vi "KE622x -- Delta Meas Example.vi"() -> ()   [LabVIEW 2010, in "Keithley 622x.lvlib"]
doc: "Example VI that shows how to perform a 'Delta' measurement. This VI requires both a 622x and a 2182/2182A nano-voltmeter."
uses:
  Keithley 622x.lvlib
  <instrlib>/Keithley 622x LV 2009/Configure/2182 -A/Low Level/Typedefs/KE2182 -- Voltage Ranges.ctl
  <instrlib>/Keithley 622x LV 2009/Configure/2182 -A/Low Level/Typedefs/KE2182 -- NPLCs.ctl
  <instrlib>/Keithley 622x LV 2009/Configure/2182 -A/Low Level/Typedefs/KE2182 -- Filter Type.ctl
  <instrlib>/Keithley 622x LV 2009/Configure/2182 -A/Low Level/Typedefs/KE2182 -- Filter Count.ctl
  <instrlib>/Keithley 622x LV 2009/Configure/2182 -A/Low Level/Typedefs/KE2182 -- Filter Window.ctl
  Configure/Delta PDelta DCon Modes/Low Level/Typedefs/KE622x -- Delta DCon Mode Delay.ctl
  Configure/Delta PDelta DCon Modes/Low Level/Typedefs/KE622x -- Delta PDelta Mode High Level.ctl
  Configure/Delta PDelta DCon Modes/Low Level/Typedefs/KE622x -- Delta PDelta Mode Low Level.ctl
  Configure/Delta PDelta DCon Modes/Low Level/Typedefs/KE622x -- Delta PDelta Mode Num Cycles.ctl
  Configure/Delta PDelta DCon Modes/Low Level/Typedefs/KE622x -- Delta PDelta Mode Num Cycles Mode.ctl
  Configure/Delta PDelta DCon Modes/Typedefs/KE622x -- Delta Mode Params.ctl
  Configure/Units/Typedefs/KE622x -- Voltage Meas Units.ctl
  Configure/Format/Typedefs/KE622x -- Optional Meas Elements.ctl
  Configure/Format/Typedefs/KE622x -- Results Format.ctl
panel:
  out "error out":errorcluster
  in  "Tab Control":enum32{"Results Table", "Plot"}(tab)
  out "Results Table":string[][](table)
  out "Plot":sgl[](graph)
  in  "Results Format":T1={"Results Format"=enum."Single Prec Bin", "Bin Byte Order"=enum."Swapped"}
  in  "Meas Elements To Return":T2={"Timstamp?"=TRUE, "Reading Num?"=TRUE, "Source Value?"=TRUE, "Compliance?"=TRUE, "Average Voltage?"=TRUE}
  out "Meas\nTimeout?":bool
  out "Execution Time\n(secs)":dbl
  in  "Meas Timeout\n(msecs)":u32=20000
  in  "Meas Units":T3=enum."Ohms"
  in  "622x Delta Meas Mode Params":T4={"High Level (A)"=0.001, "Low Level (A)"=-0.001, "Delay (s)"=0.002, "Num Cycles Mode"=enum."Finite Count", "Finite Count"=10, "Abort On\nCompliance?"=FALSE, "Cold Swithing\nMode Enabled?"=FALSE} {"Finite Count" min=2 max=65536; "Low Level (A)" min=-0.105 max=0.0 format="%.3p"; "High Level (A)" min=0.0 max=0.105 format="%.3p"; "Delay (s)" min=0.001 max=9999.999 format="%.3f"}
  in  "2182/2182A Delta Mode Meas Params":T15={"Auto Range?"=TRUE, "Man / Selected\nRange"=enum."10mV", "Enable Digital\nFilter?"=FALSE, "Filter Type"=enum."Moving", "Filter Count"=10, "Filter\nWindow (%)"=0.01, "Enable Analog\nFilter?"=FALSE, "NPLCs"=5} {"Filter\nWindow (%)" min=0.0 max=10.0 step=0.01 format="%.2f"; "Filter Count" min=1 max=100; "NPLCs" min=1 max=10}
  in  "Check For SCPI Errors? (T)":bool=TRUE
  in  "622x Resource":refnum<visa-resource-name>
  # "Input"
  # "Output"
  # "Reading Num"
  # "*** NOTE:  \"Average Voltage\"\nis only available for Differential\nConductance measurements."
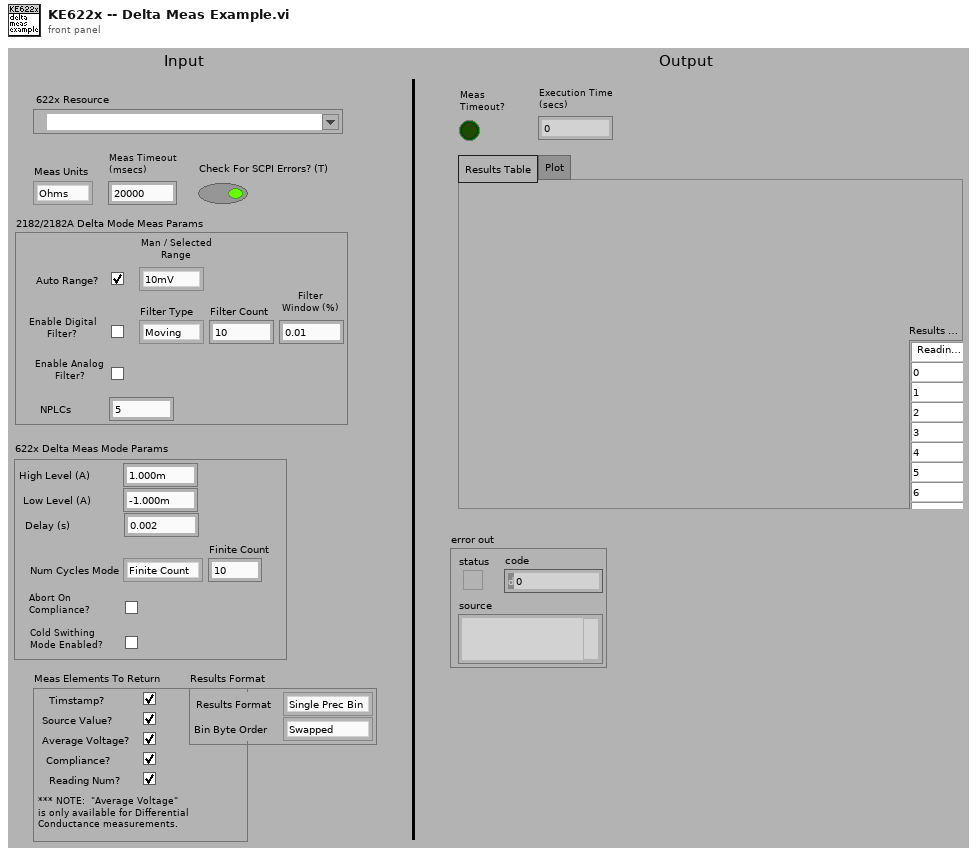
[diagram p1: front panel]
types:
  T1 = typedef "Keithley 622x.lvlib/KE622x -- Results Format.ctl" = cluster{"Results Format":enum16{"ASCII", "Single Prec Bin", "Double Prec Bin"}, "Bin Byte Order":enum16{"Normal", "Swapped"}}
  T2 = typedef "Keithley 622x.lvlib/KE622x -- Optional Meas Elements.ctl" = cluster{"Timstamp?":bool, "Reading Num?":bool, "Source Value?":bool, "Compliance?":bool, "Average Voltage?":bool}
  T3 = typedef "Keithley 622x.lvlib/KE622x -- Voltage Meas Units.ctl" = enum16{"Volts", "Ohms", "Watts", "Siemens"}
  T4 = typedef "Keithley 622x.lvlib/KE622x -- Delta Mode Params.ctl" = cluster{"High Level (A)":T5, "Low Level (A)":T6, "Delay (s)":T7, "Num Cycles Mode":T8, "Finite Count":T9, "Abort On\nCompliance?":bool, "Cold Swithing\nMode Enabled?":bool}
  T5 = typedef "Keithley 622x.lvlib/KE622x -- Delta PDelta Mode High Level.ctl" = dbl
  T6 = typedef "Keithley 622x.lvlib/KE622x -- Delta PDelta Mode Low Level.ctl" = dbl
  T7 = typedef "Keithley 622x.lvlib/KE622x -- Delta DCon Mode Delay.ctl" = dbl
  T8 = typedef "Keithley 622x.lvlib/KE622x -- Delta PDelta Mode Num Cycles Mode.ctl" = enum16{"Finite Count", "Infinite"}
  T9 = typedef "Keithley 622x.lvlib/KE622x -- Delta PDelta Mode Num Cycles.ctl" = u32
  T10 = typedef "Keithley 622x.lvlib/KE2182 -- Voltage Ranges.ctl" = enum16{"10mV", "100mV", "1V", "10V", "100V"}
  T11 = typedef "Keithley 622x.lvlib/KE2182 -- Filter Type.ctl" = enum16{"Moving", "Repeat"}
  T12 = typedef "Keithley 622x.lvlib/KE2182 -- Filter Count.ctl" = u32
  T13 = typedef "Keithley 622x.lvlib/KE2182 -- Filter Window.ctl" = dbl
  T14 = typedef "Keithley 622x.lvlib/KE2182 -- NPLCs.ctl" = u32
  T15 = cluster{"Auto Range?":bool, "Man / Selected\nRange":T10, "Enable Digital\nFilter?":bool, "Filter Type":T11, "Filter Count":T12, "Filter\nWindow (%)":T13, "Enable Analog\nFilter?":bool, "NPLCs":T14}
  T16 = typedef "Keithley 622x.lvlib/KE622x -- Trace Buf.ctl" = cluster{"Additional Valid Arrays":T2, "Reading Num":u32[], "Timestamp (secs)":sgl[], "Source Val (A)":sgl[], "Reading":sgl[], "Average Voltage (V)":sgl[], "Compliance?":bool[]}
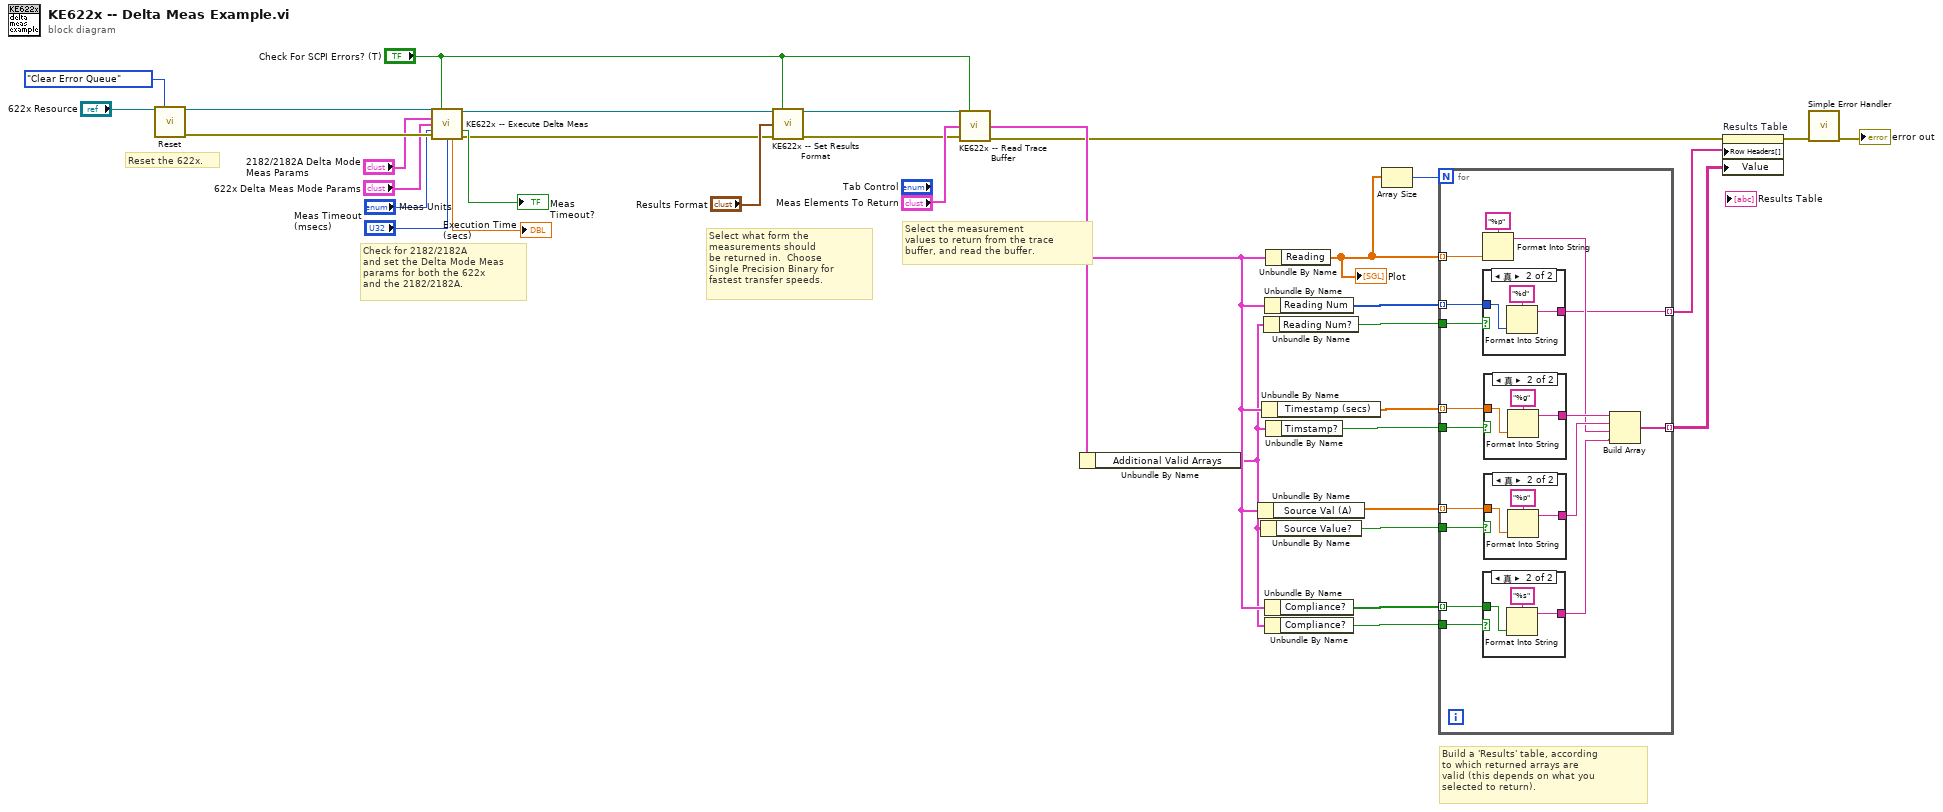
[diagram p0: block diagram]
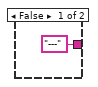
[diagram p2: hidden frame]
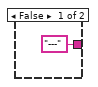
[diagram p3: hidden frame]
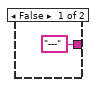
[diagram p4: hidden frame]
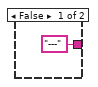
[diagram p5: hidden frame]
diagram:
  # "Build a 'Results' table, according\nto which returned arrays are\nvalid (this depends on what you\nselected to return)."
  # "Select what form the\nmeasurements should\nbe returned in.  Choose\nSingle Precision Binary for\nfastest transfer speeds."
  # "Select the measurement\nvalues to return from the trace\nbuffer, and read the buffer."
  # "Check for 2182/2182A\nand set the Delta Mode Meas\nparams for both the 622x\nand the 2182/2182A."
  # "Reset the 622x."
  n1 = call "Reset.vi"("VISA resource name"="622x Resource", "Error Queue Option"=enum16{"Clear Error Queue", "Error Query"}."Clear Error Queue") -> ("VISA resource name out"=w32:refnum<visa-resource-name>, "error out"=w31:errorcluster)  [unwired: 12 in]
  n2 = call "KE622x -- Execute Delta Meas.vi"("Resource In"=w32, "Check For SCPI Errors? (T)"="Check For SCPI Errors? (T)", "2812 -A Params In"="2182/2182A Delta Mode Meas Params", "Delta Mode Params In"="622x Delta Meas Mode Params", "Meas Units"="Meas Units", "error in (no error)"=w31, "Timeout (20000 ms)"="Meas Timeout\n(msecs)") -> ("Resource Out (dupl)"=w20:refnum<visa-resource-name>, "Timeout?"=→"Meas\nTimeout?":bool, "Execution Time"=→"Execution Time\n(secs)":dbl, "error out"=w19:errorcluster)  [unwired: 3 in, 2 out]
  n3 = call <instrlib>:"KE622x -- Set Results Format.vi"("Resource In"=w20, "Check For SCPI Errors? (T)"="Check For SCPI Errors? (T)", "Results Format"="Results Format", "error in (no error)"=w19) -> ("Resource Out (dupl)"=w23:refnum<visa-resource-name>, "error out"=w18:errorcluster)  [unwired: 10 in]
  n4 = call "KE622x -- Read Trace Buffer.vi"("Resource In"=w23, "Check For SCPI Errors? (T)"="Check For SCPI Errors? (T)", "Meas Elements To Return"="Meas Elements To Return", "error in (no error)"=w18) -> ("Trace Buf"=w10:T16, "error out"=w6:errorcluster)  [unwired: 9 in, 1 out]
  n5 = Unbundle By Name(w10) -> ("Additional Valid Arrays"=w9:T2)
  n6 = Unbundle By Name(w10) -> ("Source Val (A)"=w12:sgl[])
  n7 = Unbundle By Name(w9) -> ("Source Value?"=w11:bool)
  n8 = Unbundle By Name(w10) -> ("Timestamp (secs)"=w14:sgl[])
  n9 = Unbundle By Name(w9) -> ("Reading Num?"=w15:bool)
  n10 = Unbundle By Name(w10) -> ("Reading Num"=w16:u32[])
  n11 = Unbundle By Name(w10) -> ("Compliance?"=w8:bool[])
  n12 = Unbundle By Name(w9) -> ("Compliance?"=w7:bool)
  n13 = Unbundle By Name(w10) -> ("Reading"=w3:sgl[])
  "Plot" <- w3
  n14 = Unbundle By Name(w9) -> ("Timstamp?"=w13:bool)
  n15 = Array Size(array=w3) -> (size(s)=w17:i32)
  n16 = for {
    N: w17 -> [_]
    tunnel: w3 -> [w50] mode=indexing
    tunnel: w15 -> [w48]
    tunnel: w16 -> [w47] mode=indexing
    tunnel: w14 -> [w46] mode=indexing
    tunnel: w13 -> [w45]
    tunnel: w12 -> [w44] mode=indexing
    tunnel: w11 -> [w43]
    tunnel: w8 -> [w42] mode=indexing
    tunnel: w7 -> [w41]
    tunnel: [w36] -> w5 mode=indexing
    tunnel: [w35] -> w4 mode=indexing
    n17 = Format Into String(format string="%p", w50) -> (resulting string=w38:string)  [unwired: 2 in, 1 out]
    n18 = case shown="真" w48 {
      tunnel: w47 -> [_ w65]
      tunnel: ["---" w64] -> w36
      frame False {
      }
      frame True {
        n19 = Format Into String(format string="%d", w65) -> (resulting string=w64:string)  [unwired: 2 in, 1 out]
      }
    }
    n20 = case shown="真" w41 {
      tunnel: w42 -> [_ w53]
      tunnel: ["---" w52] -> w37
      frame False {
      }
      frame True {
        n21 = Format Into String(format string="%s", w53) -> (resulting string=w52:string)  [unwired: 2 in, 1 out]
      }
    }
    n22 = case shown="真" w45 {
      tunnel: w46 -> [_ w61]
      tunnel: ["---" w60] -> w40
      frame False {
      }
      frame True {
        n23 = Format Into String(format string="%g", w61) -> (resulting string=w60:string)  [unwired: 2 in, 1 out]
      }
    }
    n24 = case shown="真" w43 {
      tunnel: w44 -> [_ w57]
      tunnel: ["---" w56] -> w39
      frame False {
      }
      frame True {
        n25 = Format Into String(format string="%p", w57) -> (resulting string=w56:string)  [unwired: 2 in, 1 out]
      }
    }
    n26 = Build Array(w40, w39, w38, w37) -> (w35:string[])
  }
  n27 = property on="Results Table" class="Tbl (严格)"(error in=w6, "Row Headers[]"=w5, "Value"=w4) -> (error out=w2:errorcluster)  [unwired: 1 in, 1 out]
  n28 = call <vilib>:"Simple Error Handler.vi"("error in (no error)"=w2) -> ("error out"=→"error out":errorcluster)  [unwired: 4 in, 4 out]
